vi "table_number_stringI.vi"(6 "nejistota osciloskop":dbl[](array[numeric]), 7 "cislo mereni":dbl, 8 "vysledek osciloskop":dbl[](array[numeric]), 9 "nejistota citac":dbl[](array[numeric]), 10 "vysledek citac":dbl[](array[numeric]), 11 "kmitocet gen":dbl) -> (2 "Array":string[](array[string]))   [LabVIEW 2022 SP3]
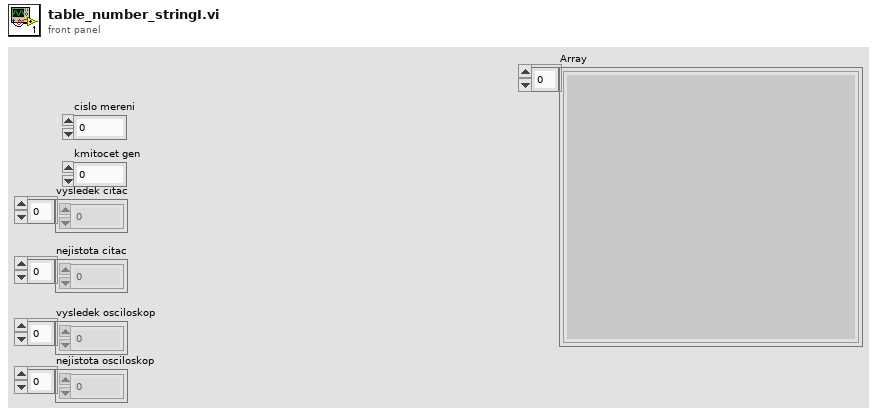
[diagram p1: front panel]
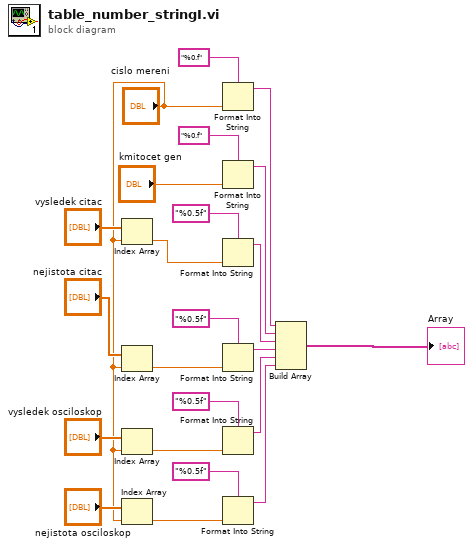
[diagram p0: block diagram]
diagram:
  n1 = Index Array(array="vysledek citac", index="cislo mereni") -> (element=w14:dbl)
  n2 = Index Array(array="nejistota citac", index="cislo mereni") -> (element=w15:dbl)
  n3 = Index Array(array="vysledek osciloskop", index="cislo mereni") -> (element=w16:dbl)
  n4 = Index Array(array="nejistota osciloskop", index="cislo mereni") -> (element=w17:dbl)
  n5 = Format Into String(format string="%0.f", "cislo mereni") -> (resulting string=w13:string)  [unwired: 2 in, 1 out]
  n6 = Format Into String(format string="%0.f", "kmitocet gen") -> (resulting string=w12:string)  [unwired: 2 in, 1 out]
  n7 = Format Into String(format string="%0.5f", w14) -> (resulting string=w11:string)  [unwired: 2 in, 1 out]
  n8 = Format Into String(format string="%0.5f", w15) -> (resulting string=w10:string)  [unwired: 2 in, 1 out]
  n9 = Format Into String(format string="%0.5f", w16) -> (resulting string=w9:string)  [unwired: 2 in, 1 out]
  n10 = Format Into String(format string="%0.5f", w17) -> (resulting string=w8:string)  [unwired: 2 in, 1 out]
  n11 = Build Array(w13, w12, w11, w10, w9, w8) -> (→"Array":string[])
